vi "fgv.vi"(8 "error in (no error)":errorcluster, 10 "Numeric in":i32, 11 "Command":T1) -> (0 "error out":errorcluster, 3 "Numeric out":i32)   [LabVIEW 2013]
uses:
  fgv.ctl
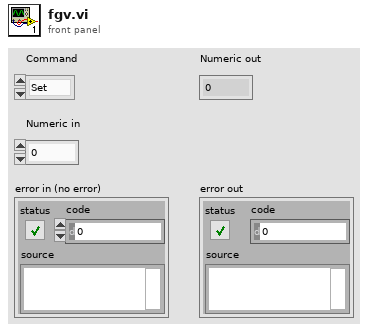
[diagram p1: front panel]
types:
  T1 = typedef "fgv.ctl" = enum16{"Set", "Get"}
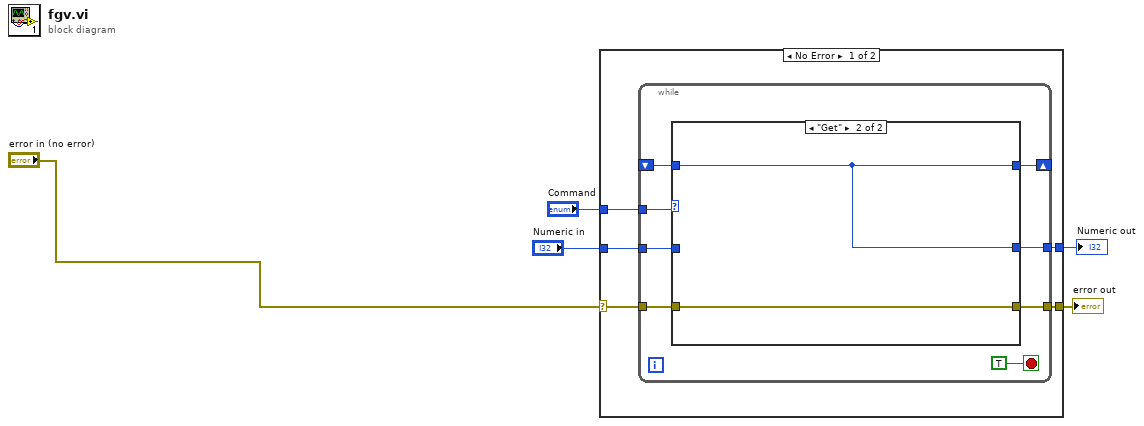
[diagram p0: block diagram]
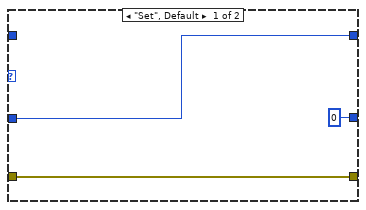
[diagram p2: hidden frame]
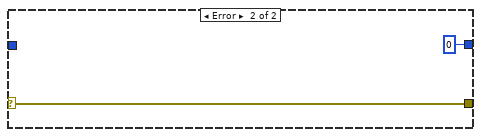
[diagram p3: hidden frame]
diagram:
  n1 = case shown="No Error" "error in (no error)" {
    selector: "error in (no error)" -> [w6 w25]
    tunnel: "Command" -> [w10 _]
    tunnel: "Numeric in" -> [w9 _]
    tunnel: [w8 0 ("Numeric")] -> w3
    tunnel: [w7 w25] -> w5
    frame No Error {
      n2 = while {
        tunnel: w10 -> [w17]
        tunnel: w9 -> [w16]
        shift-right: [w15] -> _
        shift-left: _ -> [w14]
        tunnel: [w13] -> w8
        tunnel: [w12] -> w7
        tunnel: w6 -> [w11]
        stop <- TRUE stop-if-true
        n3 = case shown="\"Get\"" w17 {
          tunnel: w16 -> [w21 _]
          tunnel: [w21 w23] -> w15
          tunnel: w14 -> [_ w23]
          tunnel: [0 ("Numeric") w23] -> w13
          tunnel: [w19 w22] -> w12
          tunnel: w11 -> [w19 w22]
          frame "Set", Default {
          }
          frame "Get" {
          }
        }
      }
    }
    frame Error {
    }
  }
  "error out" <- w5
  "Numeric out" <- w3
